vi "Eagle_FPGA Intensities Control.vi"() -> ()   [LabVIEW 2015]
uses:
  <vilib>/rvi/Emulation/niFpgaGetClockAttributes.vi
  <vilib>/rvi/Emulation/niFpgaSctlEmulationGetInTimedLoop.vi
  <vilib>/rvi/Emulation/niFpgaEmulationReportErrorSimple.vi
  <vilib>/rvi/eio/common/nirviEmuTemplateMethod_errors.vi
  <vilib>/rvi/Emulation/niFpgaCriticalErrorInLSC.vi
  <vilib>/eio/EIONode/EIONode.xnode
panel:
  in  "RB Intensity":fxp<+,16,3>
  in  "LR Intensity":fxp<+,16,3>
  in  "AB Intensity":fxp<+,16,3>
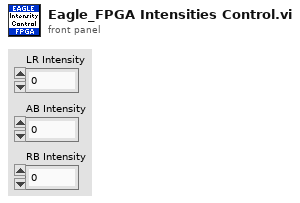
[diagram p1: front panel]
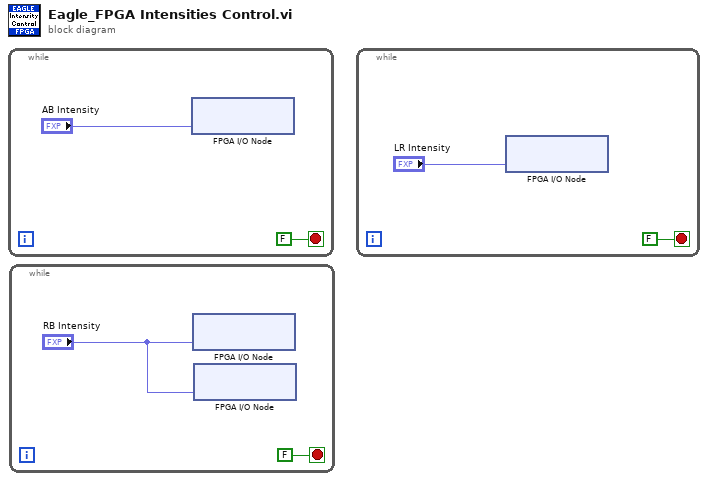
[diagram p0: block diagram]
diagram:
  n1 = while {
    stop <- FALSE stop-if-true
    n2 = xnode "FPGA I/O Node"("Mod3/AO6"="AB Intensity") -> ()  [unwired: 1 in, 1 out]
  }
  n3 = while {
    stop <- FALSE stop-if-true
    n4 = xnode "FPGA I/O Node"("Mod3/AO4"="RB Intensity") -> ()  [unwired: 1 in, 1 out]
    n5 = xnode "FPGA I/O Node"("Mod3/AO5"="RB Intensity") -> ()  [unwired: 1 in, 1 out]
  }
  n6 = while {
    stop <- FALSE stop-if-true
    n7 = xnode "FPGA I/O Node"("Mod3/AO2"="LR Intensity") -> ()  [unwired: 1 in, 1 out]
  }
